vi "grading average.vi"(10 "input array":dbl[](array[numeric])) -> (2 "avg":dbl)   [LabVIEW 2019]
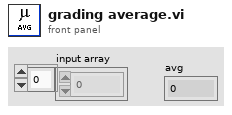
[diagram p1: front panel]
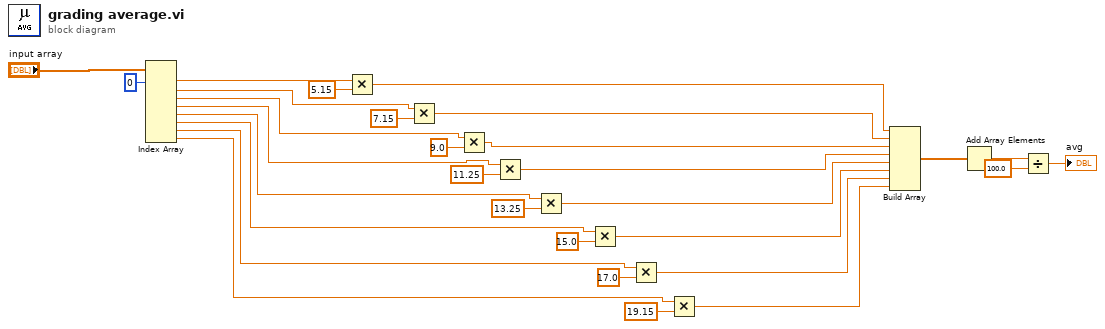
[diagram p0: block diagram]
diagram:
  n1 = Index Array(array="input array", index #1=0 ("index")) -> (element #1=w28:dbl, element #2=w25:dbl, element #3=w23:dbl, element #4=w21:dbl, element #5=w19:dbl, element #6=w17:dbl, element #7=w15:dbl, element #8=w13:dbl)  [unwired: 7 in]
  n2 = Multiply(x=w28, y=5.15) -> (x*y=w12:dbl)
  n3 = Multiply(x=w25, y=7.15) -> (x*y=w11:dbl)
  n4 = Multiply(x=w23, y=9.0) -> (x*y=w10:dbl)
  n5 = Multiply(x=w21, y=11.25) -> (x*y=w9:dbl)
  n6 = Multiply(x=w19, y=13.25) -> (x*y=w8:dbl)
  n7 = Multiply(x=w17, y=15.0) -> (x*y=w7:dbl)
  n8 = Multiply(x=w15, y=17.0) -> (x*y=w6:dbl)
  n9 = Multiply(x=w13, y=19.15) -> (x*y=w5:dbl)
  n10 = Build Array(w12, w11, w10, w9, w8, w7, w6, w5) -> (w4:dbl[])
  n11 = Add Array Elements(numeric array=w4) -> (sum=w3:dbl)
  n12 = Divide(x=w3, y=100.0) -> (x/y=→"avg":dbl)
